vi "PKG_IMC_GetADdata.vi"(9 "ch":i32, 10 "ADdata":dbl, 11 "handle":u32) -> (1 "function return":i32, 2 "ADdata out":dbl, 3 "handle out":u32)   [LabVIEW 2011, in "IMC_Pkg4xxx.lvlib"]
doc: "PKG_IMC_GetADdata(IMC_HANDLE handle, double *ADdata, int ch);"
uses:
  IMC_Pkg4xxx.lvlib
  IMC_Pkg4xxx.dll
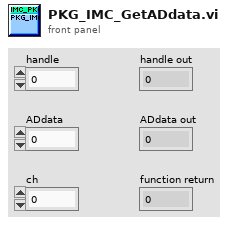
[diagram p1: front panel]
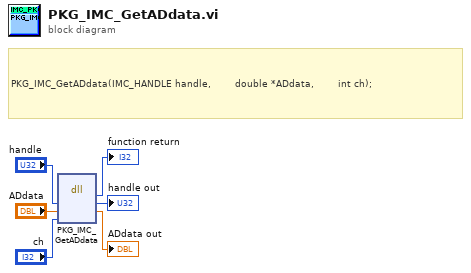
[diagram p0: block diagram]
diagram:
  # "PKG_IMC_GetADdata(IMC_HANDLE handle, \t\t \t\t\t\tdouble *ADdata,\t\t\t\t\t\t\t\tint ch);"
  n1 = dll-call lib="PTH1mabs F光盘刻录\niMC MotionIMCNet_V4.0IMCAppincLabviewIMC_PKG4xxxIMC_PKG4xxx\nIMC_Pkg4xxx.*" fn="PKG_IMC_GetADdata"("handle"="handle", "ADdata"="ADdata", "ch"="ch") -> (→"function return":i32, "handle"=→"handle out":u32, "ADdata"=→"ADdata out":dbl)  [unwired: 4 in, 2 out]
